vi "New LINX SPI Channel.vi"(8 "error in (no error)":errorcluster, 10 "CS Configuration":T1, 11 "LINX Resource":T3) -> (0 "error out":errorcluster, 3 "LINX SPI out":refnum<class "LINX SPI.lvclass">)   [LabVIEW 2020, in "LINX SPI.lvclass"]
uses:
  LINX SPI.lvclass
  <vilib>/MakerHub/LINX/Private/Type Defs/LINX Ref.ctl
  <vilib>/MakerHub/LINX/LMH-LINX.lvlib
  <vilib>/MakerHub/LINX/Private/Type Defs/Platform.ctl
  <vilib>/MakerHub/LINX/Private/Type Defs/Interface.ctl
  <vilib>/MakerHub/LINX/Private/Device/Type Defs/LINX Device Config.ctl
  <vilib>/MakerHub/LINX/Private/Device/Device.lvlib
  <vilib>/MakerHub/LINX/Private/Device/Type Defs/TCP Config.ctl
  <vilib>/MakerHub/LINX/Private/Device/Type Defs/Channels.ctl
  <vilib>/MakerHub/LINX/Private/Type Defs/Peripherals/SPI/SPI CS Logic Level.ctl
  <vilib>/MakerHub/LINX/Public/Peripherals/SPI/SPI CS Config.ctl
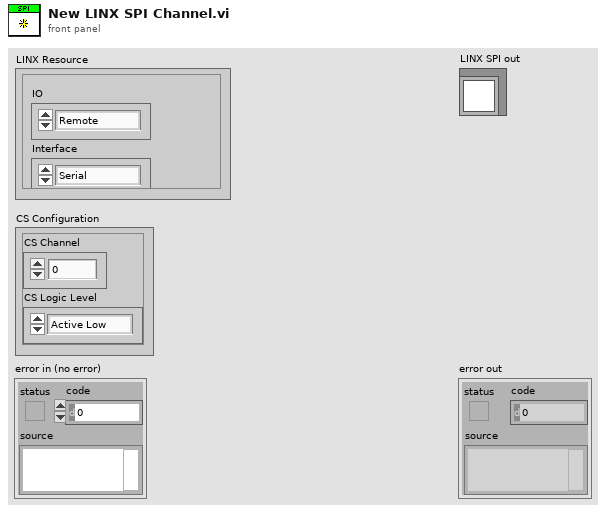
[diagram p1: front panel]
types:
  T1 = typedef "LMH-LINX.lvlib/SPI CS Config.ctl" = cluster{"CS Channel":u8, "CS Logic Level":T2}
  T2 = typedef "LMH-LINX.lvlib/SPI CS Logic Level.ctl" = enum8{"Active Low", "Active High"}
  T3 = typedef "LMH-LINX.lvlib/LINX Ref.ctl" = cluster{"IO":T4, "Interface":T5, "LINX Device Config":T6}
  T4 = typedef "LMH-LINX.lvlib/Platform.ctl" = enum16{"Remote", "Local"}
  T5 = typedef "LMH-LINX.lvlib/Interface.ctl" = enum16{"Serial", "TCP"}
  T6 = typedef "LMH-LINX.lvlib/Device.lvlib/LINX Device Config.ctl" = cluster{"Interface":T5, "COM Port":refnum<visa-resource-name>, "TCP Configuration":T7, "Device Family":u8, "Device ID":u8, "Device Name":string, "TCP Ref":refnum<k5>, "Channels":T8}
  T7 = typedef "LMH-LINX.lvlib/Device.lvlib/TCP Config.ctl" = cluster{"IP Address":string, "Port":u16}
  T8 = typedef "LMH-LINX.lvlib/Channels.ctl" = cluster{"DI":u8[], "DO":u8[], "AI":u8[], "AO":u8[], "PWM":u8[], "QE":u8[], "UART":u8[], "I2C 2":u8[], "SPI":u8[], "CAN":u8[], "Servo":u8[], "AI Ref (V)":dbl, "AI Resolution (Bits)":u8, "AO Ref (V)":dbl, "AO Resolution (Bits)":u8}
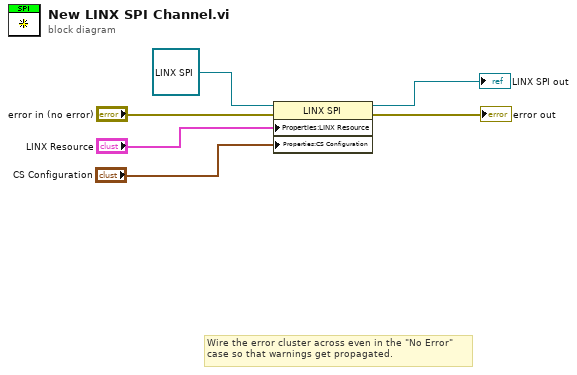
[diagram p0: block diagram]
diagram:
  # "Wire the error cluster across even in the \"No Error\"\ncase so that warnings get propagated."
  n1 = property class="LINX SPI"(reference=refnum<class "LINX SPI.lvclass"> refnum ("LINX SPI in"), error in="error in (no error)", "Properties:LINX Resource"="LINX Resource", "Properties:CS Configuration"="CS Configuration") -> (reference out=→"LINX SPI out":refnum<class "LINX SPI.lvclass">, error out=→"error out":errorcluster)
